vi "Shooter VI.vi"() -> ()   [LabVIEW 2016]
uses:
  <vilib>/Rock Robotics/WPI/MotorControl/WPI_MotorControlDeviceRef.ctl
  <vilib>/Rock Robotics/WPI/MotorControl/WPI_MotorControlType.ctl
  <vilib>/Rock Robotics/SystemInterfaces/DIO/FPGA_DIOPWMChannel.ctl
  <vilib>/Rock Robotics/WPI/PWM/WPI_PWMDeadband.ctl
panel:
  in  "bottomWheelMotor":T1={"DeviceStatus"={"status"=FALSE, "code"=0, "source"=""}, "Type"=enum."PWM", "PWM"={"PWM Channel"=enum."Invalid", "DeadBand"={"Name"="", "maxPositivePwm"=0, "minPositivePwm"=0, "centerPwm"=0, "maxNegativePwm"=0, "minNegativePwm"=0, "angularRange"=0}}, "CAN"={"Device Number"=0, "SetOutput VI Ref"=variant(enum8{"Percent VBus", "Current", "Speed", "Position", "Voltage"} enum."Percent VBus"), "GetOutput VI Ref"=variant(refnum<k1> refnum), "Enable VI Ref"=variant(dbl 12.0), "Disable VI Ref"=variant(enum8{"Percent VBus", "Speed", "Position", "Slave", "Unchanged / Invalid"} enum."Percent VBus"), "Data"=variant}, "Invert"=FALSE}
  in  "topWheelMotor":T1={"DeviceStatus"={"status"=FALSE, "code"=0, "source"=""}, "Type"=enum."PWM", "PWM"={"PWM Channel"=enum."Invalid", "DeadBand"={"Name"="", "maxPositivePwm"=0, "minPositivePwm"=0, "centerPwm"=0, "maxNegativePwm"=0, "minNegativePwm"=0, "angularRange"=0}}, "CAN"={"Device Number"=0, "SetOutput VI Ref"=variant(enum8{"Percent VBus", "Current", "Speed", "Position", "Voltage"} enum."Percent VBus"), "GetOutput VI Ref"=variant(refnum<k1> refnum), "Enable VI Ref"=variant(dbl 12.0), "Disable VI Ref"=variant(enum8{"Percent VBus", "Speed", "Position", "Slave", "Unchanged / Invalid"} enum."Percent VBus"), "Data"=variant}, "Invert"=FALSE}
  out "done":bool
  in  "bottomWheel":T5
  in  "topWheel":T6
  in  "bottomInvert":bool
  in  "topInvert":bool
  in  "RpmStableVal":dbl
  in  "RpmThreshold":dbl
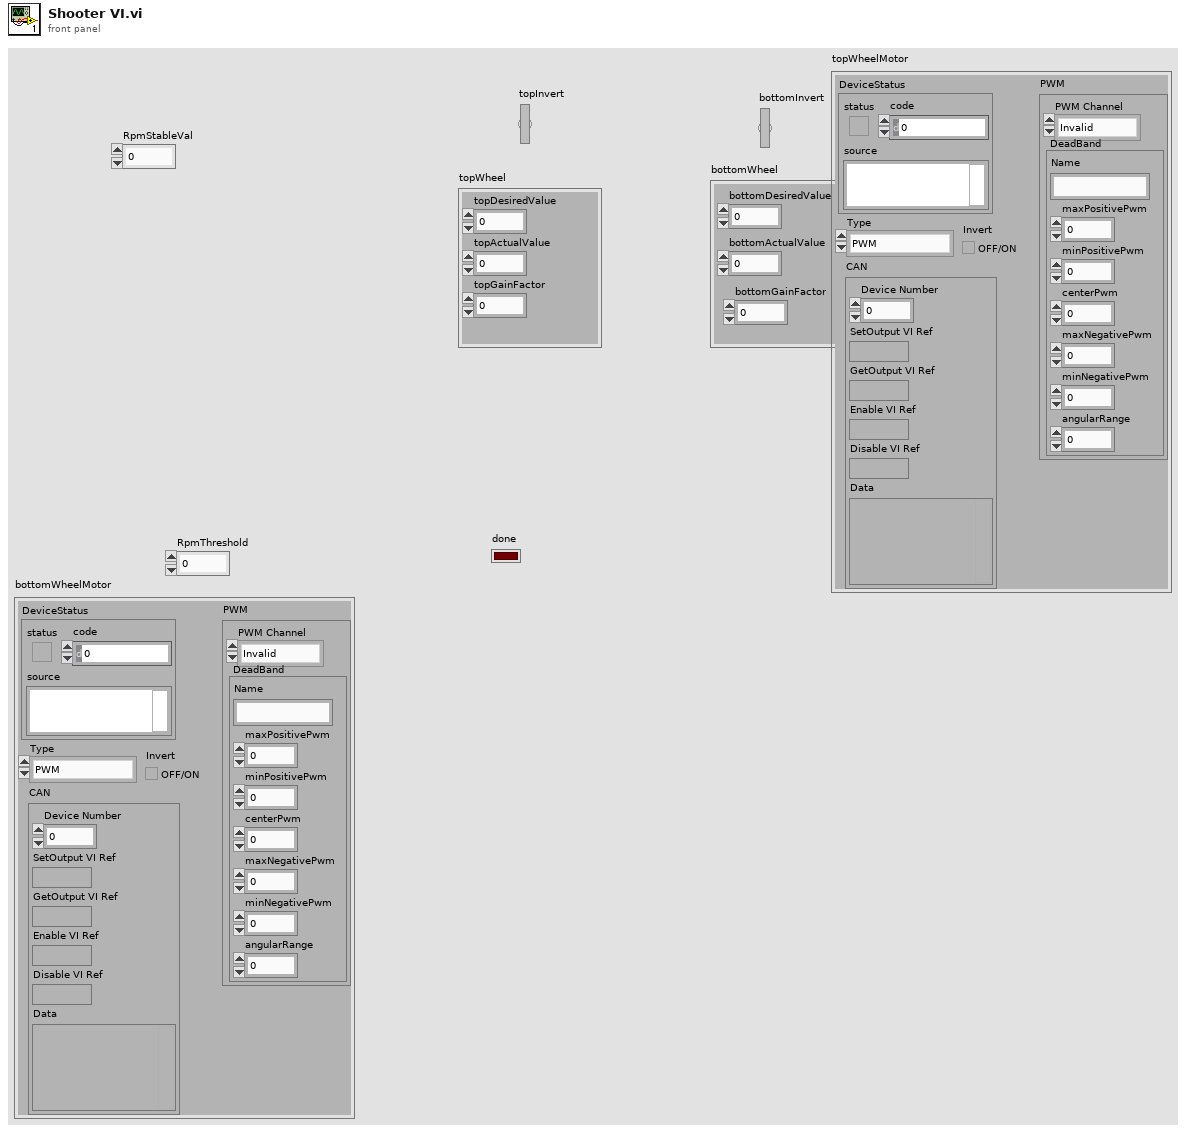
[diagram p1: front panel]
types:
  T1 = typedef "WPI_MotorControlDeviceRef.ctl" = cluster{"DeviceStatus":errorcluster, "Type":T2, "PWM":cluster{"PWM Channel":T3, "DeadBand":T4}, "CAN":cluster{"Device Number":u8, "SetOutput VI Ref":variant, "GetOutput VI Ref":variant, "Enable VI Ref":variant, "Disable VI Ref":variant, "Data":variant}, "Invert":bool}
  T2 = typedef "WPI_MotorControlType.ctl" = enum16{"PWM", "CAN"}
  T3 = typedef "FPGA_DIOPWMChannel.ctl" = enum8{"PWM 0", "PWM 1", "PWM 2", "PWM 3", "PWM 4", "PWM 5", "PWM 6", "PWM 7", "PWM 8", "PWM 9", "PWM MXP 0", "PWM MXP 1", "PWM MXP 2", "PWM MXP 3", "PWM MXP 4", "PWM MXP 5", "PWM MXP 6", "PWM MXP 7", "PWM MXP 8", "PWM MXP 9", "Invalid"}
  T4 = typedef "WPI_PWMDeadband.ctl" = cluster{"Name":string, "maxPositivePwm":i32, "minPositivePwm":i32, "centerPwm":i32, "maxNegativePwm":i32, "minNegativePwm":i32, "angularRange":u16}
  T5 = cluster{"bottomDesiredValue":dbl, "bottomActualValue":dbl, "bottomGainFactor":dbl}
  T6 = cluster{"topDesiredValue":dbl, "topActualValue":dbl, "topGainFactor":dbl}
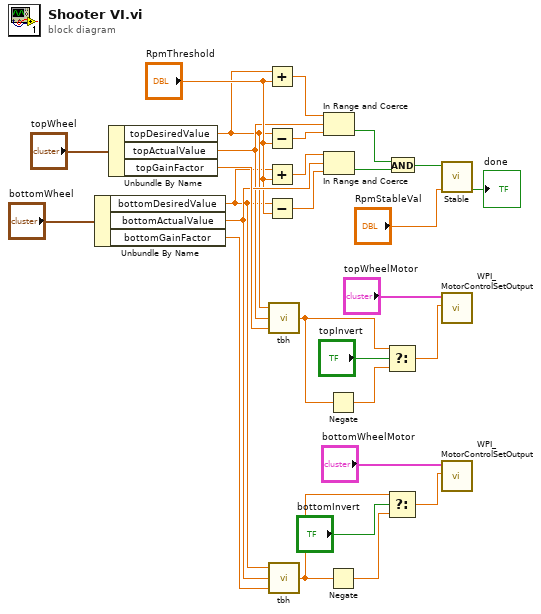
[diagram p0: block diagram]
diagram:
  n1 = Unbundle By Name("bottomWheel") -> ("bottomDesiredValue"=w6:dbl, "bottomActualValue"=w14:dbl, "bottomGainFactor"=w17:dbl)
  n2 = Unbundle By Name("topWheel") -> ("topDesiredValue"=w7:dbl, "topActualValue"=w8:dbl, "topGainFactor"=w19:dbl)
  n3 = Add(x=w7, y="RpmThreshold") -> (x+y=w10:dbl)
  n4 = Subtract(x=w7, y="RpmThreshold") -> (x-y=w11:dbl)
  n5 = Add(x=w6, y="RpmThreshold") -> (x+y=w16:dbl)
  n6 = Subtract(x=w6, y="RpmThreshold") -> (x-y=w15:dbl)
  n7 = call <userlib>:"tbh.vi"("Gain Factor"=w19, "Actual Value"=w8, "Desired Value"=w7) -> ("Out"=w26:dbl)
  n8 = call <userlib>:"tbh.vi"("Gain Factor"=w17, "Actual Value"=w14, "Desired Value"=w6) -> ("Out"=w21:dbl)
  n9 = In Range and Coerce(upper limit=w10, x=w8, lower limit=w11) -> (In Range?=w12:bool)  [unwired: 1 out]
  n10 = In Range and Coerce(upper limit=w16, x=w14, lower limit=w15) -> (In Range?=w13:bool)  [unwired: 1 out]
  n11 = Negate(x=w26) -> (-x=w25:dbl)
  n12 = Negate(x=w21) -> (-x=w22:dbl)
  n13 = Select(t=w26, s="topInvert", f=w25) -> (s? t:f=w27:dbl)
  n14 = Select(t=w21, s="bottomInvert", f=w22) -> (s? t:f=w23:dbl)
  n15 = And(x=w12, y=w13) -> (x .and. y?=w3:bool)
  n16 = call <userlib>:"Stable.vi"("Eval Period (sec)"="RpmStableVal", "Signal Input"=w3) -> ("Stable"=→"done":bool)  [unwired: 9 in]
  n17 = call <vilib>:"WPI_MotorControlSetOutput.vi"("Output"=w27, "MotorControlDevRef"="topWheelMotor") -> ()  [unwired: 7 in, 3 out]
  n18 = call <vilib>:"WPI_MotorControlSetOutput.vi"("Output"=w23, "MotorControlDevRef"="bottomWheelMotor") -> ()  [unwired: 7 in, 3 out]
